vi "Get Printf Event.vi"(8 "error in (no error)":errorcluster) -> (0 "error out":errorcluster, 1 "Verbose Level":i32, 2 "stdout event":refnum<user-event>)   [LabVIEW 2013, in "SET_Printf.lvlib" / "LV_Printf Core.lvclass"]
uses:
  LV_Printf Core.lvclass
  Messages/General/LV_Printf Msg.lvclass
  LV_Printf Core.lvclass/LV_Printf Core.ctl
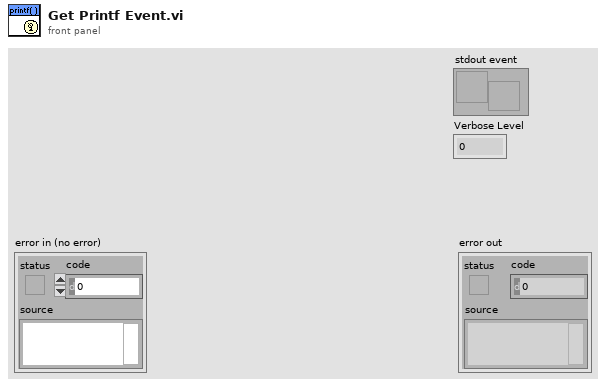
[diagram p1: front panel]
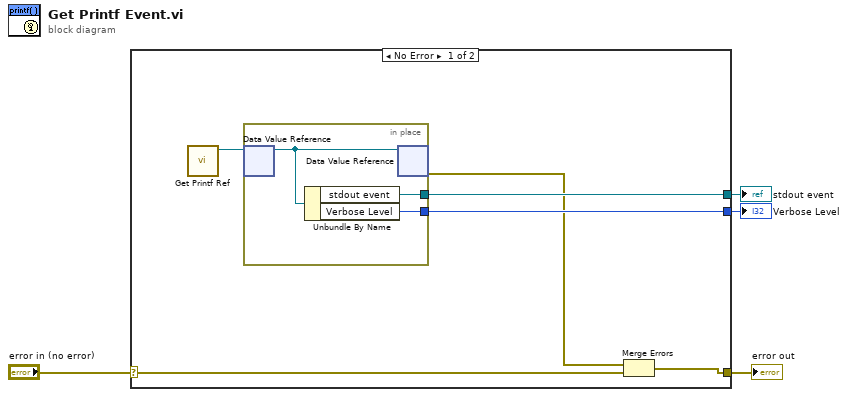
[diagram p0: block diagram]
diagram:
  n1 = case shown="No Error" "error in (no error)" {
    selector: "error in (no error)" -> [w7 w14]
    tunnel: [w5 w14] -> w3
    tunnel: [w9 _] -> w2
    tunnel: [w8 _] -> w1
    frame No Error {
      n2 = call "Get Printf Ref.vi"() -> ("Printf DVR"=w10:refnum<data-value>)  [unwired: 11 in]
      n3 = in-place {
        in-place-border: [w12] -> w9
        in-place-border: [w11] -> w8
        n4 = in-place-dvr #1(w10) -> (w13:refnum<class "LV_Printf Core.lvclass">)  [unwired: 1 out]
        n5 = Unbundle By Name(w13) -> ("stdout event"=w12:refnum<user-event>, "Verbose Level"=w11:i32)
        n6 = in-place-dvr #1(w13) -> (w6:errorcluster)  [unwired: 1 out]
      }
      n7 = Merge Errors(w6, w7) -> (w5:errorcluster)
    }
    frame Error {
    }
  }
  "error out" <- w3
  "stdout event" <- w2
  "Verbose Level" <- w1
